vi "get_bounding_box.vi"(8 "error in (no error)":errorcluster, 11 "GenericTrajectory in":refnum<class "GenericTrajectory.lvclass">) -> (0 "error out":errorcluster, 2 "Box.lvclass":refnum<class "Box.lvclass">, 3 "GenericTrajectory out":refnum<class "GenericTrajectory.lvclass">)   [LabVIEW 2010, in "GenericTrajectory.lvclass"]
uses:
  GenericTrajectory.lvclass
  common/classes/Box/Box/Box.lvclass
  GenericTrajectory.lvclass/GenericTrajectory.ctl
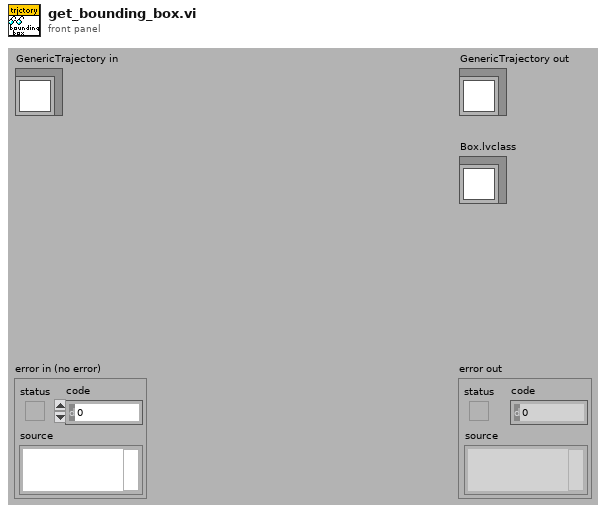
[diagram p1: front panel]
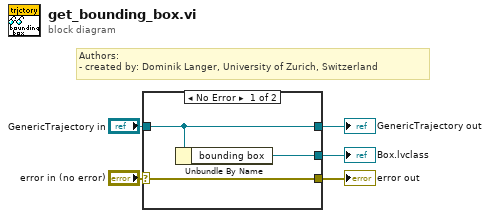
[diagram p0: block diagram]
diagram:
  # "Authors: \n- created by: Dominik Langer, University of Zurich, Switzerland"
  n1 = case shown="No Error" "error in (no error)" {
    selector: "error in (no error)" -> [w8 w9]
    tunnel: [w8 w9] -> w4
    tunnel: [w7 w10] -> w2
    tunnel: "GenericTrajectory in" -> [w7 w10]
    tunnel: [w6 _] -> w1
    frame No Error {
      n2 = Unbundle By Name(w7) -> ("bounding box"=w6:refnum<class "Box.lvclass">)
    }
    frame Error {
    }
  }
  "error out" <- w4
  "GenericTrajectory out" <- w2
  "Box.lvclass" <- w1
